vi "qTCI.vi"(0 "System no.":i32=1 min=1 max=4 step=1, 1 "Board":i32=1 min=1 max=10 step=1, 5 "error in":errorcluster) -> (14 "Calculated analog value":dbl format="%.6f", 19 "error out":errorcluster)   [LabVIEW 2026]
doc: "Queries calculated fast alignment input value. Answer is TAV? value calculated with method set by SIC. \n\nC-887, E-712, E-727.AS:"
panel:
  # "Queries Calculated fast alignment Input value. Answer is TAV? Value calculated with method set by SIC."
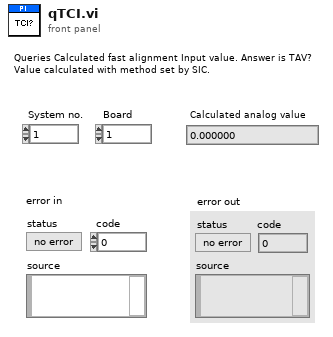
[diagram p1: front panel]
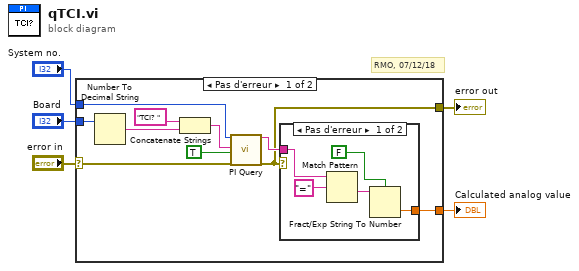
[diagram p0: block diagram]
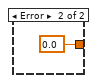
[diagram p2: hidden frame]
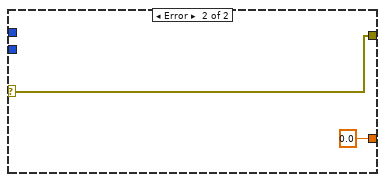
[diagram p3: hidden frame]
diagram:
  # "RMO, 07/12/18"
  n1 = case shown="Pas d'erreur" "error in" {
    selector: "error in" -> [w9 w23]
    tunnel: [w6 w23] -> w5
    tunnel: "Board" -> [w14 _]
    tunnel: "System no." -> [w12 _]
    tunnel: [w10 0.0] -> w2
    frame No Error {
      n2 = Number To Decimal String(number=w14) -> (decimal integer string=w11:string)  [unwired: 1 out]
      n3 = Concatenate Strings("TCI? ", w11) -> (w13:string)
      n4 = call "PI Query.vi"("System no."=w12, "String to send"=w13, "Attach termination char.?"=TRUE ("Attach Linefeed?"), "error in"=w9) -> ("String read"=w7:string, "error out"=w6:errorcluster)  [unwired: 3 in, 11 out]
      n5 = case shown="Pas d'erreur" w6 {
        tunnel: w7 -> [w20 _]
        tunnel: [w19 0.0] -> w10
        frame No Error {
          n6 = Match Pattern(string=w20, regular expression="=") -> (after substring=w17:string)  [unwired: 4 out]
          n7 = Fract/Exp String To Number(use system decimal point (T)=FALSE, string=w17) -> (number=w19:dbl)  [unwired: 3 out]
        }
        frame Error {
        }
      }
    }
    frame Error {
    }
  }
  "error out" <- w5
  "Calculated analog value" <- w2
